vi "CTL_Limit Check.vi"(8 "E-Stop":bool, 9 "Limit":dbl, 11 "X":dbl) -> (1 "X< Neg":bool, 2 "Neg <X<Pos":bool, 3 "X>Pos":bool)   [LabVIEW 2024]
doc: "X>Pos is TRUE if the X is greater than Pos Limit\nX<Pos is TRUE if the X is Less than Neg Limit\nNeg <X< Pos is TRUE when X is between the two limits"
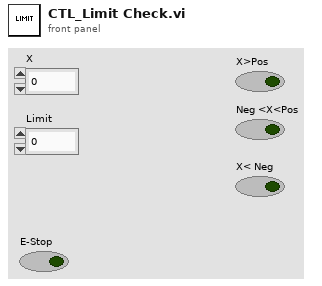
[diagram p1: front panel]
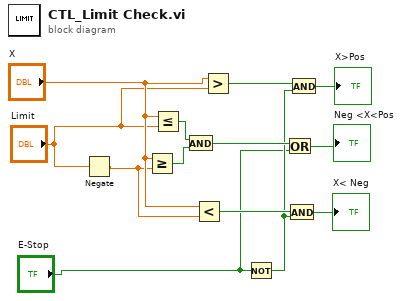
[diagram p0: block diagram]
diagram:
  n1 = Negate(x="Limit") -> (-x=w1:dbl)
  n2 = Greater Or Equal?(x="X", y=w1) -> (x >= y?=w12:bool)
  n3 = Less Or Equal?(x="X", y="Limit") -> (x <= y?=w13:bool)
  n4 = And(x=w13, y=w12) -> (x .and. y?=w6:bool)
  n5 = Less?(x="X", y=w1) -> (x < y?=w7:bool)
  n6 = Greater?(x="X", y="Limit") -> (0:w5:bool)
  n7 = Not(x="E-Stop") -> (.not. x?=w4:bool)
  n8 = Or(x=w6, y="E-Stop") -> (x .or. y?=→"Neg <X<Pos":bool)
  n9 = And(x=w7, y=w4) -> (x .and. y?=→"X< Neg":bool)
  n10 = And(x=w5, y=w4) -> (x .and. y?=→"X>Pos":bool)
